vi "Read IPS PSU Current Voltage.vi"(6 "PSU #":i32=1 min=1 max=6, 8 "error in (no error)":errorcluster, 11 "Instrument.OxfordVRM in":refnum<class "Instrument.OxfordVRM.lvclass">) -> (0 "error out":errorcluster, 1 "Voltage (V)":dbl, 2 "Current (A)":dbl, 3 "Instrument.OxfordVRM out":refnum<class "Instrument.OxfordVRM.lvclass">)   [LabVIEW 2019, in "Instrument.OxfordVRM.lvclass"]
uses:
  Instrument.OxfordVRM.lvclass
  Instrument.OxfordVRM.lvclass/Instrument.OxfordVRM.ctl
  <instrlib>/Mercury iXX/Public/Libraries/Magnet/Open/Open Magnet Device.vi
  <instrlib>/Mercury iXX/Public/Libraries/Magnet/Signals/Read/Current (Read).vi
  <instrlib>/Mercury iXX/Public/Libraries/Magnet/Signals/Read/Voltage (Read).vi
  <instrlib>/Mercury iXX/Mercury iXX.lvlib
  <instrlib>/Mercury iXX/Public/Libraries/Magnet.lvlib
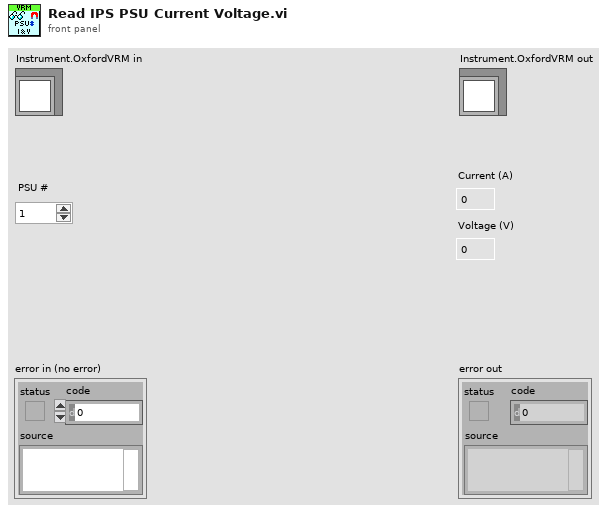
[diagram p1: front panel]
types:
  T1 = typedef "Mercury iXX.lvlib/Mercury Reference.ctl" = cluster{"Comms":refnum<visa-resource-name>, "Device ID":string[], "Comms Layer":T2, "Command":string, "Query reference":T3}
  T2 = typedef "Mercury iXX.lvlib/Comms Transport Layer.ctl" = enum16{"Ethernet TCP/IP", "USB", "ISOBus - RS-232", "GPIB"}
  T3 = typedef "Mercury iXX.lvlib/Query Dynamic Reference.ctl" = refnum<vi>
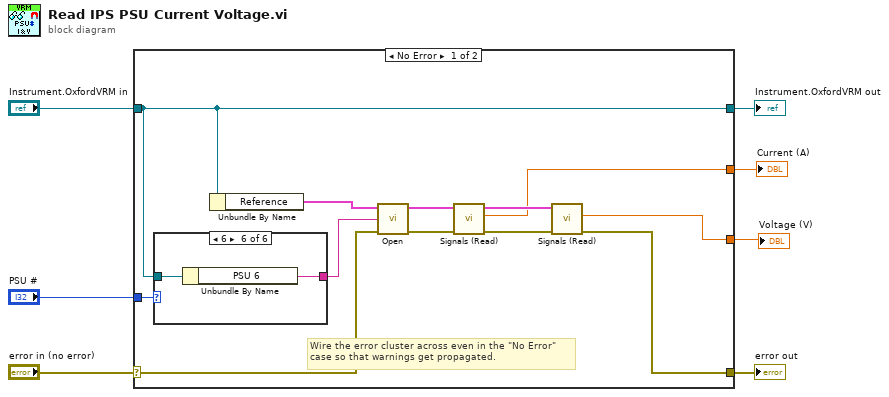
[diagram p0: block diagram]
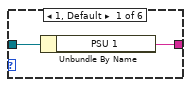
[diagram p2: hidden frame]
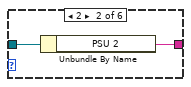
[diagram p3: hidden frame]
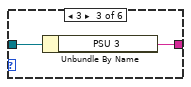
[diagram p4: hidden frame]
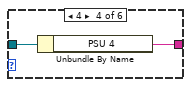
[diagram p5: hidden frame]
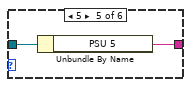
[diagram p6: hidden frame]
diagram:
  n1 = case shown="No Error" "error in (no error)" {
    selector: "error in (no error)" -> [w16 w33]
    tunnel: [w11 w33] -> w6
    tunnel: [w9 w32] -> w4
    tunnel: "Instrument.OxfordVRM in" -> [w9 w32]
    tunnel: [w12 _] -> w3
    tunnel: [w13 _] -> w2
    tunnel: "PSU #" -> [w10 _]
    frame No Error {
      # "Wire the error cluster across even in the \"No Error\"\ncase so that warnings get propagated."
      n2 = case shown="6" w10 {
        tunnel: [w21 w23 w24 w26 w28 w30] -> w8
        tunnel: w9 -> [w20 w22 w25 w27 w29 w31]
        frame 1, Default {
          n3 = Unbundle By Name(w20) -> ("PSU 1"=w21:string)
        }
        frame 2 {
          n4 = Unbundle By Name(w22) -> ("PSU 2"=w23:string)
        }
        frame 3 {
          n5 = Unbundle By Name(w25) -> ("PSU 3"=w24:string)
        }
        frame 4 {
          n6 = Unbundle By Name(w27) -> ("PSU 4"=w26:string)
        }
        frame 5 {
          n7 = Unbundle By Name(w29) -> ("PSU 5"=w28:string)
        }
        frame 6 {
          n8 = Unbundle By Name(w31) -> ("PSU 6"=w30:string)
        }
      }
      n9 = Unbundle By Name(w9) -> ("Reference"=w17:T1)
      n10 = call-poly <instrlib>:"Open.vi"("error in (no error)"=w16, "Device Identifier"=w8, "Mercury Reference In"=w17) -> ("error out"=w19:errorcluster, "Mercury Reference Out"=w18:T1)  [unwired: 7 out]
      n11 = call-poly <instrlib>:"Signals (Read).vi"("error in"=w19, "Mercury Reference In"=w18) -> ("error out"=w15:errorcluster, "Current"=w12:dbl, "Mercury Reference Out"=w14:T1)  [unwired: 1 in, 6 out]
      n12 = call-poly <instrlib>:"Signals (Read).vi"("error in"=w15, "Mercury Reference In"=w14) -> ("error out"=w11:errorcluster, "Voltage"=w13:dbl)  [unwired: 1 in, 7 out]
    }
    frame Error {
    }
  }
  "error out" <- w6
  "Instrument.OxfordVRM out" <- w4
  "Current (A)" <- w3
  "Voltage (V)" <- w2
